vi "Display Confirmation to User.vi"(6 "Calling VI in":refnum<vi>, 7 "Confirmation Type":T6, 8 "error in (no error)":errorcluster, 11 "Config":T2) -> (0 "error out":errorcluster, 1 "New Config?":bool, 2 "Which Button?":T1(ring), 3 "Config out":T2)   [LabVIEW 2020, in "VI Properties Editor.lvlib"]
doc: "Displays a confirmation dialog to the user, taking into account <B>Confirmation Type</B> and <B>Config</B>."
uses:
  VI Properties Editor.lvlib
  CTLs/Confirmation Type.ctl
  CTLs/Config.ctl
  CTLs/Filter Info.ctl
  CTLs/Filter Column.ctl
  CTLs/Filter Type.ctl
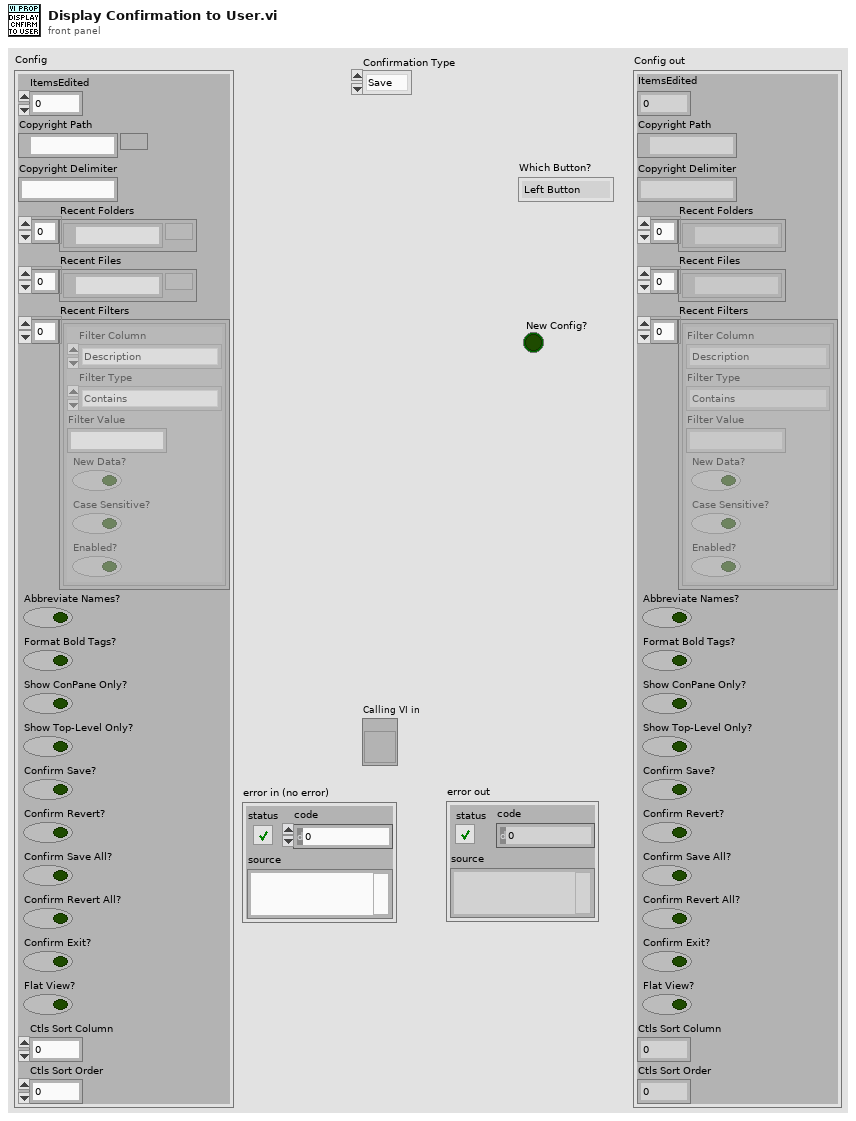
[diagram p1: front panel]
types:
  T1 = enum16{"Left Button", "Center Button", "Right Button", "Window Close"}
  T2 = typedef "VI Properties Editor.lvlib/Config.ctl" = cluster{"ItemsEdited":u32, "Copyright Path":path, "Copyright Delimiter":string, "Recent Folders":path[], "Recent Files":path[], "Recent Filters":T3[], "Abbreviate Names?":bool, "Format Bold Tags?":bool, "Show ConPane Only?":bool, "Show Top-Level Only?":bool, "Confirm Save?":bool, "Confirm Revert?":bool, "Confirm Save All?":bool, "Confirm Revert All?":bool, "Confirm Exit?":bool, "Flat View?":bool, "Ctls Sort Column":i32, "Ctls Sort Order":i32}
  T3 = typedef "VI Properties Editor.lvlib/Filter Info.ctl" = cluster{"Filter Column":T4, "Filter Type":T5, "Filter Value":string, "New Data?":bool, "Case Sensitive?":bool, "Enabled?":bool}
  T4 = typedef "VI Properties Editor.lvlib/Filter Column.ctl" = enum16{"Name", "Path", "Type", "Window Title", "Description", "Help Path", "Help Tag", "Custom Title?", "Reentrancy", "Inlined?", "Help URL", "Help Type", "Allow Debugging?", "Auto Error Handling?", "Run When Opened?", "Suspend When Called?", "Priority", "Preferred Exec Sytem", "Control Label", "Control Caption", "Control Description", "Control Tip Strip"}
  T5 = typedef "VI Properties Editor.lvlib/Filter Type.ctl" = enum16{"Contains", "Equals", "Starts with", "Ends with", "Is empty", "Does not contain", "Does not equal", "Is not empty"}
  T6 = typedef "VI Properties Editor.lvlib/Confirmation Type.ctl" = enum16{"Save", "Revert", "Save All", "Revert All", "Exit"}
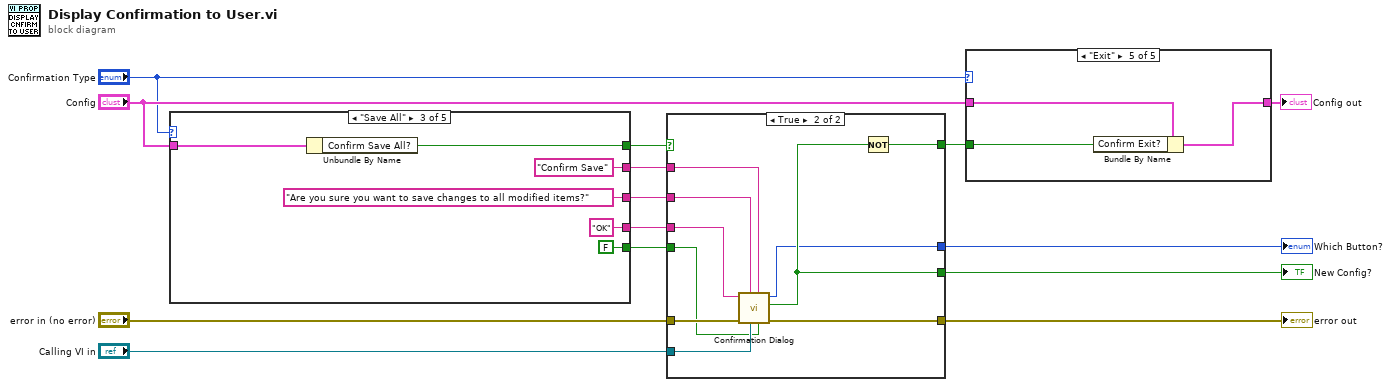
[diagram p0: block diagram]
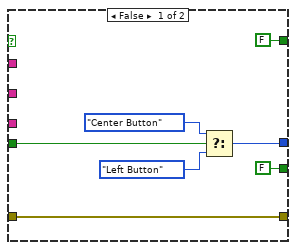
[diagram p2: hidden frame]
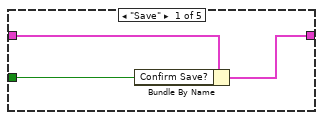
[diagram p3: hidden frame]
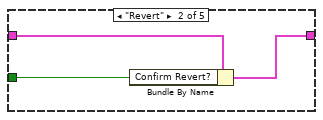
[diagram p4: hidden frame]
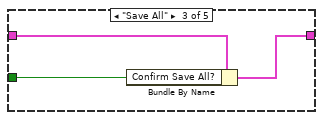
[diagram p5: hidden frame]
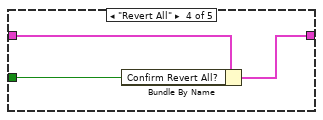
[diagram p6: hidden frame]
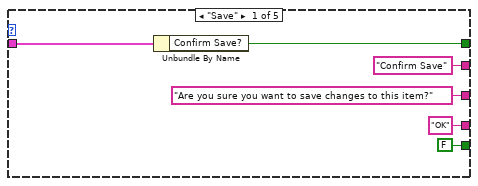
[diagram p7: hidden frame]
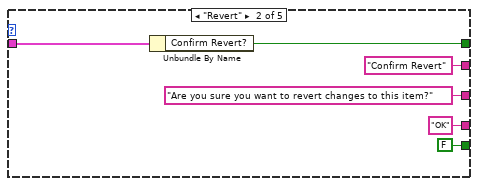
[diagram p8: hidden frame]
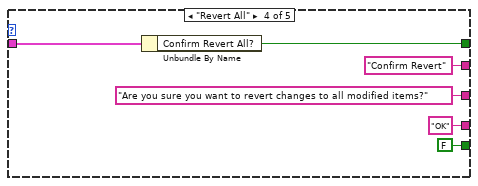
[diagram p9: hidden frame]
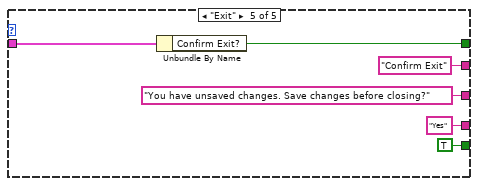
[diagram p10: hidden frame]
diagram:
  n1 = case shown="\"Save All\"" "Confirmation Type" {
    tunnel: ["Are you sure you want to save changes to this item?" "Are you sure you want to revert changes to this item?" "Are you sure you want to save changes to all modified items?" "Are you sure you want to revert changes to all modified items?" "You have unsaved changes. Save changes before closing?"] -> w11
    tunnel: "Config" -> [w19 w25 w31 w37 w43]
    tunnel: [w18 w24 w30 w36 w42] -> w6
    tunnel: ["Confirm Save" "Confirm Revert" "Confirm Save" "Confirm Revert" "Confirm Exit"] -> w14
    tunnel: ["OK" "OK" "OK" "OK" "Yes"] -> w2
    tunnel: [FALSE FALSE FALSE FALSE TRUE] -> w1
    frame "Save" {
      n2 = Unbundle By Name(w19) -> ("Confirm Save?"=w18:bool)
    }
    frame "Revert" {
      n3 = Unbundle By Name(w25) -> ("Confirm Revert?"=w24:bool)
    }
    frame "Save All" {
      n4 = Unbundle By Name(w31) -> ("Confirm Save All?"=w30:bool)
    }
    frame "Revert All" {
      n5 = Unbundle By Name(w37) -> ("Confirm Revert All?"=w36:bool)
    }
    frame "Exit" {
      n6 = Unbundle By Name(w43) -> ("Confirm Exit?"=w42:bool)
    }
  }
  n7 = case shown="True" w6 {
    tunnel: w14 -> [_ w55]
    tunnel: "error in (no error)" -> [w50 w61]
    tunnel: [w50 w60] -> w12
    tunnel: w11 -> [_ w54]
    tunnel: [FALSE w57] -> w7
    tunnel: [FALSE w58] -> w5
    tunnel: "Calling VI in" -> [_ w59]
    tunnel: [w45 w56] -> w3
    tunnel: w2 -> [_ w53]
    tunnel: w1 -> [w48 w52]
    frame False {
      n8 = Select(t=T1."Center Button" ("Which Button?"), s=w48, f=T1."Left Button" ("Which Button?")) -> (s? t:f=w45:T1)
    }
    frame True {
      n9 = call "Confirmation Dialog.vi"("Middle Button Visible?"=w52, "Window Title (\"\")"=w55, "Calling VI in"=w59, "Message"=w54, "error in (no error)"=w61, "Left Button Text (\"OK\")"=w53) -> ("error out"=w60:errorcluster, "Skip Prompts?"=w57:bool, "Which Button?"=w56:T1)  [unwired: 3 in]
      n10 = Not(x=w57) -> (.not. x?=w58:bool)
    }
  }
  "error out" <- w12
  "New Config?" <- w7
  "Which Button?" <- w3
  n11 = case shown="\"Exit\"" "Confirmation Type" {
    tunnel: "Config" -> [w64 w67 w70 w73 w76]
    tunnel: [w63 w66 w69 w72 w75] -> w8
    tunnel: w5 -> [w62 w65 w68 w71 w74]
    frame "Save" {
      n12 = Bundle By Name(cluster=w64, "Confirm Save?"=w62) -> (w63:T2)
    }
    frame "Revert" {
      n13 = Bundle By Name(cluster=w67, "Confirm Revert?"=w65) -> (w66:T2)
    }
    frame "Save All" {
      n14 = Bundle By Name(cluster=w70, "Confirm Save All?"=w68) -> (w69:T2)
    }
    frame "Revert All" {
      n15 = Bundle By Name(cluster=w73, "Confirm Revert All?"=w71) -> (w72:T2)
    }
    frame "Exit" {
      n16 = Bundle By Name(cluster=w76, "Confirm Exit?"=w74) -> (w75:T2)
    }
  }
  "Config out" <- w8
